vi "Primes.vi"(1 "Number":i32) -> (0 "Prime Factors":i32)   [LabVIEW 2016]
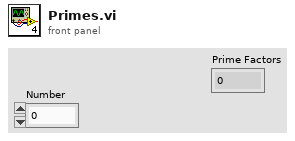
[diagram p1: front panel]
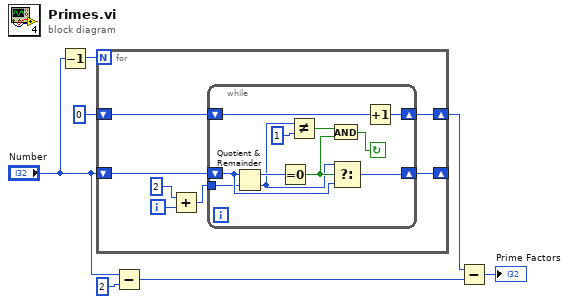
[diagram p0: block diagram]
diagram:
  n1 = Decrement(x="Number") -> (x-1=w6:i32)
  n2 = for {
    N: w6 -> [_]
    shift-right: [w12] -> w5
    shift-left: 0 -> [w13]
    shift-right: [w8] -> _
    shift-left: "Number" -> [w14]
    i -> [w11]
    n3 = Add(x=2, y=w11) -> (x+y=w9:i32)
    n4 = while {
      tunnel: w9 -> [w17]
      shift-right: [w15] -> w12
      shift-left: w13 -> [w16]
      shift-right: [w18] -> w8
      shift-left: w14 -> [w20]
      stop <- w23 continue-if-true
      n5 = Quotient & Remainder(x=w20, y=w17) -> (x-y*floor(x/y)=w22:i32, floor(x/y)=w19:i32)
      n6 = Equal To 0?(x=w22) -> (x = 0?=w21:bool)
      n7 = Not Equal?(x=w19, y=1) -> (x != y?=w24:bool)
      n8 = And(x=w24, y=w21) -> (x .and. y?=w23:bool)
      n9 = Select(t=w19, s=w21, f=w20) -> (s? t:f=w18:i32)
      n10 = Increment(x=w16) -> (x+1=w15:i32)
    }
  }
  n11 = Subtract(x="Number", y=2) -> (x-y=w2:i32)
  n12 = Subtract(x=w5, y=w2) -> (x-y=→"Prime Factors":i32)
